vi "PH_BackreflectionMeas.set i Attr.vi"(0 "i ref in":refnum<vi>, 5 "error in (no error)":errorcluster) -> (14 "i ref out":refnum<vi>, 16 "i Attributes":T1={"GUI Refs"={"Get Data"=refnum, "BR State"=refnum, "Reset warning"=refnum, "Low Energy Graph"=refnum}, "Status"={"Reset Warning"=FALSE}, "Default Low Energy Chan Settings"={"Channel Name"="CH1", "Input Impedance"="MEG", "Max Input Frequency"="TWENTY", "Vertical Coupling"=1, "Channel Enabled"=TRUE, "Probe Attenuation"=1.0, "Vertical Range"=100.0, "Vertical Offset"=0.0}, "Default High Energy Chan Settings"={"Channel Name"="CH1", "Input Impedance"="MEG", "Max Input Frequency"="TWENTY", "Vertical Coupling"=1, "Channel Enabled"=TRUE, "Probe Attenuation"=1.0, "Vertical Range"=100.0, "Vertical Offset"=0.0}, "Default Trigger Settings"={"Source"="CH1", "Slope"=0, "Level [V]"=0.0}, "Default Acqu Settings"={"Time base"=2e-07, "Record Length"=10000, "Start Time"=0.0, "Type"=0, "Continuous"=FALSE}, "Limit [V]"=0.0} {"Default Acqu Settings"."Start Time" format="%#_12p"; "Default Acqu Settings"."Record Length" items=["500"=500, "10000"=10000]; "Default Acqu Settings"."Time base" items=["2ns"=2e-09, "4ns"=4e-09, "10ns"=1e-08, "20ns"=2e-08, "40ns"=4e-08, "100ns"=1e-07, "200ns"=2e-07, "400ns"=4e-07, "1µs"=1e-06, "2µs"=2e-06, "4µs"=4e-06, "10µs"=1e-05, "20µs"=2e-05, "40µs"=4e-05, "100µs"=0.0001, "200µs"=0.0002, "400µs"=0.0004, "1ms"=0.001, "2ms"=0.002, "10ms"=0.01, "20ms"=0.02, "40ms"=0.04, "100ms"=0.1, "200ms"=0.2, "400ms"=0.4, "1s"=1.0, "2s"=2.0, "4s"=4.0, "10s"=10.0]; "Default Trigger Settings"."Level [V]" format="%#_6p"; "Default High Energy Chan Settings"."Vertical Offset" format="%#_6p"; "Default High Energy Chan Settings"."Vertical Range" items=["1mV"=0.001, "2mV"=0.002, "5mV"=0.005, "10mV"=0.01, "20mV"=0.02, "50mV"=0.05, "100mV"=0.1, "200mV"=0.2, "500mV"=0.5, "1V"=1.0]; "Default High Energy Chan Settings"."Probe Attenuation" format="%#.2f"; "Default Low Energy Chan Settings"."Vertical Offset" format="%#_6p"; "Default Low Energy Chan Settings"."Vertical Range" items=["1mV"=0.001, "2mV"=0.002, "5mV"=0.005, "10mV"=0.01, "20mV"=0.02, "50mV"=0.05, "100mV"=0.1, "200mV"=0.2, "500mV"=0.5, "1V"=1.0]; "Default Low Energy Chan Settings"."Probe Attenuation" format="%#.2f"}, 19 "error out":errorcluster)   [LabVIEW 2014, in "PH_BackreflectionMeas.lvlib"]
doc: "This VI reads information from the database and writes it to own attributes."
uses:
  PH_BackreflectionMeas.lvlib
  PH_BackreflectionMeas.i attribute.ctl
  PH_TKTDS-30xx/PH_TKTDS-30xx.Channel Config.ctl
  PH_TKTDS-30xx/PH_TKTDS-30xx.Trigger Config.ctl
  PH_TKTDS-30xx/PH_TKTDS-30xx.Acquisition Config.ctl
  PH_TKTDS-30xx/PH_TKTDS-30xx.lvlib
  PH_Common/PH_Common.lvlib
  CSCore/CSSystem/CSSystemLib/CSSystemLib.lvlib
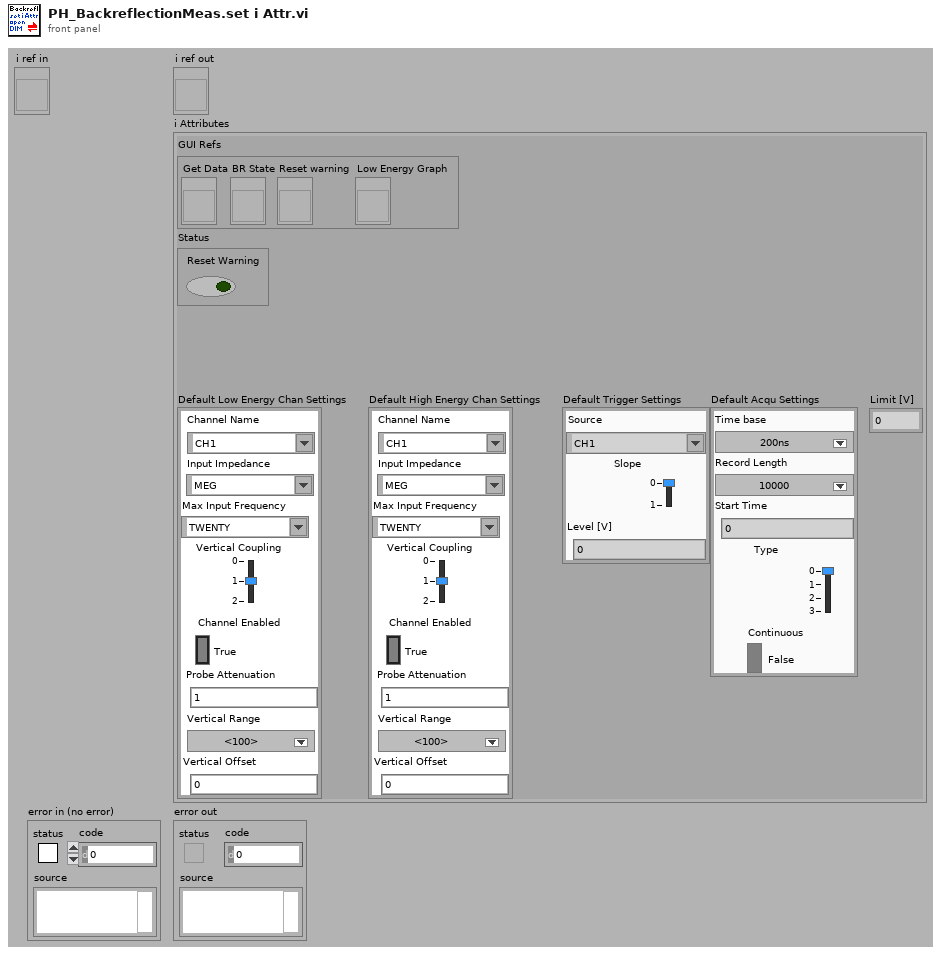
[diagram p1: front panel]
types:
  T1 = typedef "PH_BackreflectionMeas.lvlib/PH_BackreflectionMeas.i attribute.ctl" = cluster{"GUI Refs":cluster{"Get Data":refnum<vi>, "BR State":refnum<vi>, "Reset warning":refnum<vi>, "Low Energy Graph":refnum<vi>}, "Status":cluster{"Reset Warning":bool}, "Default Low Energy Chan Settings":T2, "Default High Energy Chan Settings":T2, "Default Trigger Settings":T3, "Default Acqu Settings":T4, "Limit [V]":dbl}
  T2 = typedef "PH_TKTDS-30xx.lvlib/PH_TKTDS-30xx.Channel Config.ctl" = cluster{"Channel Name":string, "Input Impedance":string, "Max Input Frequency":string, "Vertical Coupling":i32, "Channel Enabled":bool, "Probe Attenuation":dbl, "Vertical Range":dbl, "Vertical Offset":dbl}
  T3 = typedef "PH_TKTDS-30xx.lvlib/PH_TKTDS-30xx.Trigger Config.ctl" = cluster{"Source":string, "Slope":i32, "Level [V]":dbl}
  T4 = typedef "PH_TKTDS-30xx.lvlib/PH_TKTDS-30xx.Acquisition Config.ctl" = cluster{"Time base":dbl, "Record Length":u16, "Start Time":dbl, "Type":i32, "Continuous":bool}
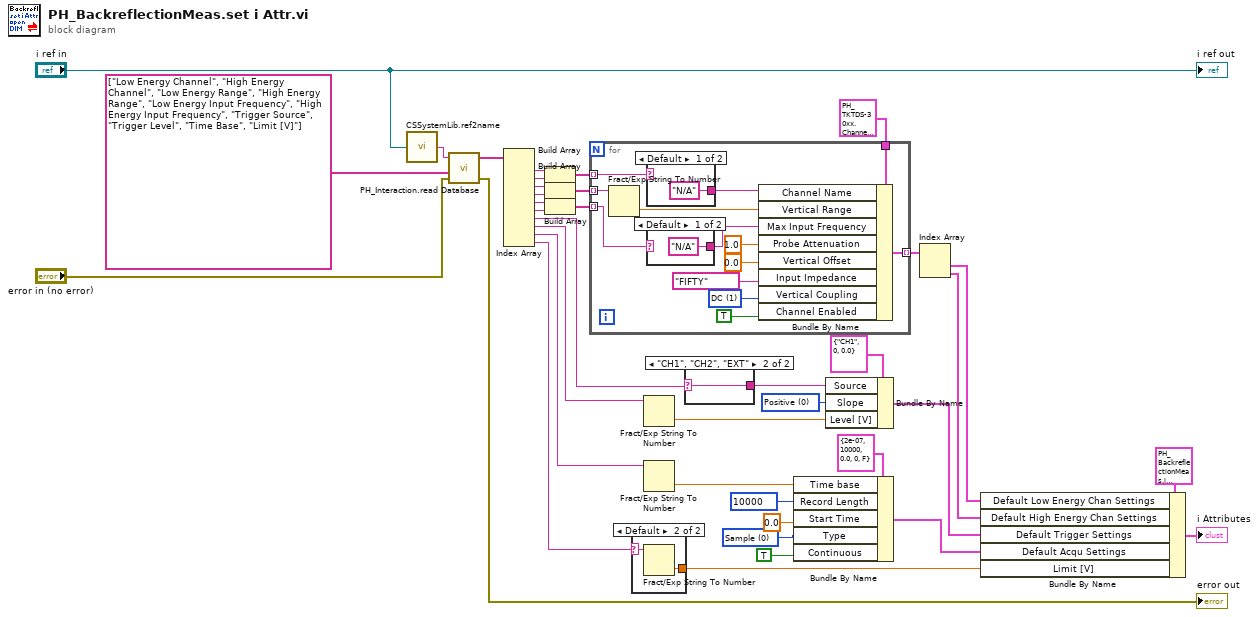
[diagram p0: block diagram]
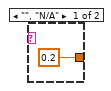
[diagram p2: hidden frame]
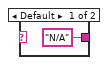
[diagram p5: hidden frame]
diagram:
  w30 = 0 items=["Sample", "Peak Detect", "Envelope", "Average"] ("Type")
  w31 = u16 10000 items=["500"=500, "10000"=10000] ("Record Length")
  w35 = 0 items=["Positive", "Negative"] ("Slope")
  n1 = call "CSSystemLib.ref2name.vi"("obj refnum"="i ref in") -> ("name"=w19:string)
  n2 = call "PH_Interaction.read Database.vi"("error in (no error)"="error in (no error)", "Strings to search for"=string[] ["Low Energy Channel", "High Energy Channel", "Low Energy Range", "High Energy Range", "Low Energy Input Frequency", "High Energy Input Frequency", "Trigger Source", "Trigger Level", "Time Base", "Limit [V]"], "DB Entry to read"=w19) -> ("error out"=→"error out":errorcluster, "Values"=w16:string[])  [unwired: 1 in]
  n3 = Index Array(array=w16) -> (element #1=w17:string, element #2=w15:string, element #3=w14:string, element #4=w13:string, element #5=w12:string, element #6=w11:string, element #7=w7:string, element #8=w6:string, element #9=w4:string, element #10=w3:string)  [unwired: 10 in]
  n4 = Build Array(w17, w15) -> (w10:string[])
  n5 = Build Array(w14, w13) -> (w9:string[])
  n6 = Build Array(w12, w11) -> (w8:string[])
  n7 = for {
    tunnel: T2 {"Channel Name"="CH1", "Input Impedance"="MEG", "Max Input Frequency"="TWENTY", "Vertical Coupling"=1, "Channel Enabled"=TRUE, "Probe Attenuation"=1.0, "Vertical Range"=100.0, "Vertical Offset"=0.0} ("Channel Sets") -> [w51]
    tunnel: [w43] -> w27 mode=indexing
    tunnel: w10 -> [w41] mode=indexing
    tunnel: w9 -> [w42] mode=indexing
    tunnel: w8 -> [w40] mode=indexing
    w48 = 1 items=["AC", "DC", "GND"] ("Vertical Coupling (DC)")
    n8 = Fract/Exp String To Number(string=w42) -> (number=w39:dbl)  [unwired: 3 in, 1 out]
    n9 = case shown="Default" w41 {
      selector: w41 -> [_ w55]
      tunnel: ["N/A" w55] -> w50
      frame Default {
      }
      frame "CH1", "CH2" {
      }
    }
    n10 = case shown="Default" w40 {
      selector: w40 -> [_ w53]
      tunnel: ["N/A" w53] -> w49
      frame Default {
      }
      frame "FULL", "ONEFIFTY", "TWENTY" {
      }
    }
    n11 = Bundle By Name(cluster=w51, "Channel Name"=w50, "Vertical Range"=w39, "Max Input Frequency"=w49, "Probe Attenuation"=1.0, "Vertical Offset"=0.0, "Input Impedance"="FIFTY" ("Input Impedance (1.0 mega ohm)"), "Vertical Coupling"=w48, "Channel Enabled"=TRUE ("Channel Enabled (True)")) -> (w43:T2)
  }
  n12 = case shown="Default" w3 {
    selector: w3 -> [_ w57]
    tunnel: [0.2 w58] -> w20
    frame "", "N/A" {
    }
    frame Default {
      n13 = Fract/Exp String To Number(string=w57) -> (number=w58:dbl)  [unwired: 3 in, 1 out]
    }
  }
  n14 = Fract/Exp String To Number(string=w6) -> (number=w5:dbl)  [unwired: 3 in, 1 out]
  n15 = Fract/Exp String To Number(string=w4) -> (number=w33:dbl)  [unwired: 3 in, 1 out]
  n16 = case shown="\"CH1\", \"CH2\", \"EXT\"" w7 {
    selector: w7 -> [_ w60]
    tunnel: ["N/A" ("Packed Settings\nChannel::Range::Input Frequency") w60] -> w36
    frame Default {
    }
    frame "CH1", "CH2", "EXT" {
    }
  }
  n17 = Bundle By Name(cluster=T4 {"Time base"=2e-07, "Record Length"=10000, "Start Time"=0.0, "Type"=0, "Continuous"=FALSE} ("Acqu Sets"), "Time base"=w33, "Record Length"=w31, "Start Time"=0.0, "Type"=w30, "Continuous"=TRUE) -> (w21:T4)
  n18 = Bundle By Name(cluster=T3 {"Source"="CH1", "Slope"=0, "Level [V]"=0.0} ("Trigger Sets"), "Source"=w36, "Slope"=w35, "Level [V]"=w5) -> (w22:T3)
  n19 = Index Array(array=w27) -> (element #1=w24:T2, element #2=w23:T2)  [unwired: 2 in]
  n20 = Bundle By Name(cluster=T1 {"GUI Refs"={"Get Data"=refnum, "BR State"=refnum, "Reset warning"=refnum, "Low Energy Graph"=refnum}, "Status"={"Reset Warning"=FALSE}, "Default Low Energy Chan Settings"={"Channel Name"="", "Input Impedance"="", "Max Input Frequency"="", "Vertical Coupling"=0, "Channel Enabled"=FALSE, "Probe Attenuation"=0.0, "Vertical Range"=0.0, "Vertical Offset"=0.0}, "Default High Energy Chan Settings"={"Channel Name"="", "Input Impedance"="", "Max Input Frequency"="", "Vertical Coupling"=0, "Channel Enabled"=FALSE, "Probe Attenuation"=0.0, "Vertical Range"=0.0, "Vertical Offset"=0.0}, "Default Trigger Settings"={"Source"="", "Slope"=0, "Level [V]"=0.0}, "Default Acqu Settings"={"Time base"=0.0, "Record Length"=0, "Start Time"=0.0, "Type"=0, "Continuous"=FALSE}, "Limit [V]"=0.0} ("CLASS.i attribute"), "Default Low Energy Chan Settings"=w24, "Default High Energy Chan Settings"=w23, "Default Trigger Settings"=w22, "Default Acqu Settings"=w21, "Limit [V]"=w20) -> (→"i Attributes":T1)
  "i ref out" <- "i ref in"
